vi "LVUT Global 1.vi"() -> ()   [LabVIEW 2019, in "Unit Test Engine Tools.lvlib"]
uses:
  Unit Test Engine Tools.lvlib
panel:
  in  "UpDataResult writer endpoint 4":refnum<k21>
  in  "UpDataResult writer endpoint 3":refnum<k21>
  in  "UpDataResult writer endpoint 2":refnum<k21>
  in  "UpDataResult writer endpoint 1":refnum<k21>
  in  "NewTests writer endpoint 4":refnum<k21>
  in  "NewTests writer endpoint 3":refnum<k21>
  in  "NewTests writer endpoint 2":refnum<k21>
  in  "NewTests writer endpoint 1":refnum<k21>
  in  "Error writer endpoint 4":refnum<k21>
  in  "Error writer endpoint 3":refnum<k21>
  in  "Error writer endpoint 2":refnum<k21>
  in  "Error writer endpoint 1":refnum<k21>
  in  "UploadSerialNumber writer endpoint 4":refnum<k21>
  in  "UploadSerialNumber writer endpoint 3":refnum<k21>
  in  "UploadSerialNumber writer endpoint 2":refnum<k21>
  in  "UploadSerialNumber writer endpoint 1":refnum<k21>
  in  "Limit Path":path
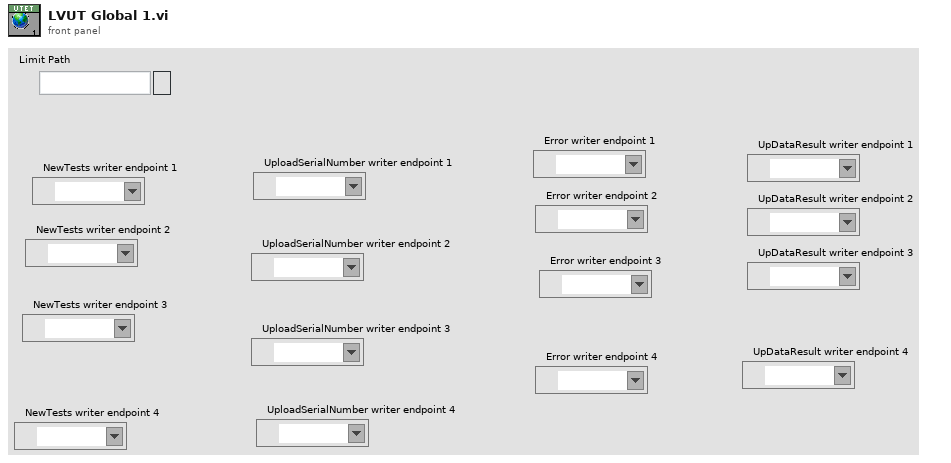
[diagram p1: front panel]
diagram:
